vi "Read Recordset (STRING).vi"(8 "error in (no error)":errorcluster, 9 "Max Rows to Fetch (-1 = all)":i32=-1, 11 "Recordset In":refnum<k7>) -> (0 "error out":errorcluster, 1 "Rows Returned":i32, 2 "Data out":string[][](array[string]), 3 "Recordset Out":refnum<k7>, 4 "Field Names":string[](array[string]))   [LabVIEW 2014, in "hse-db.lvlib" / "ADO-DB-Driver.lvlib"]
uses:
  ADO-DB-Driver.lvlib
panel:
  out "records read so far":i32
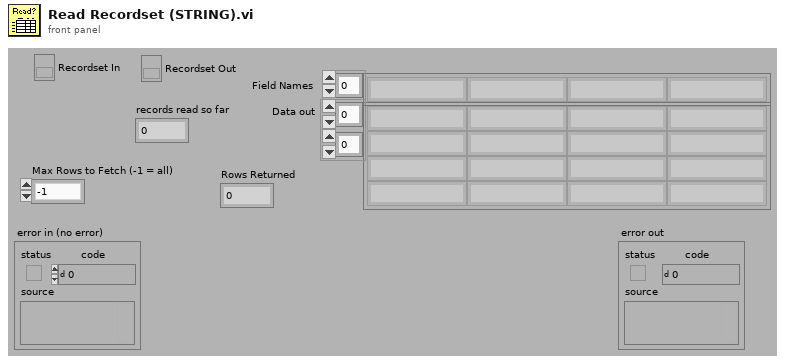
[diagram p1: front panel]
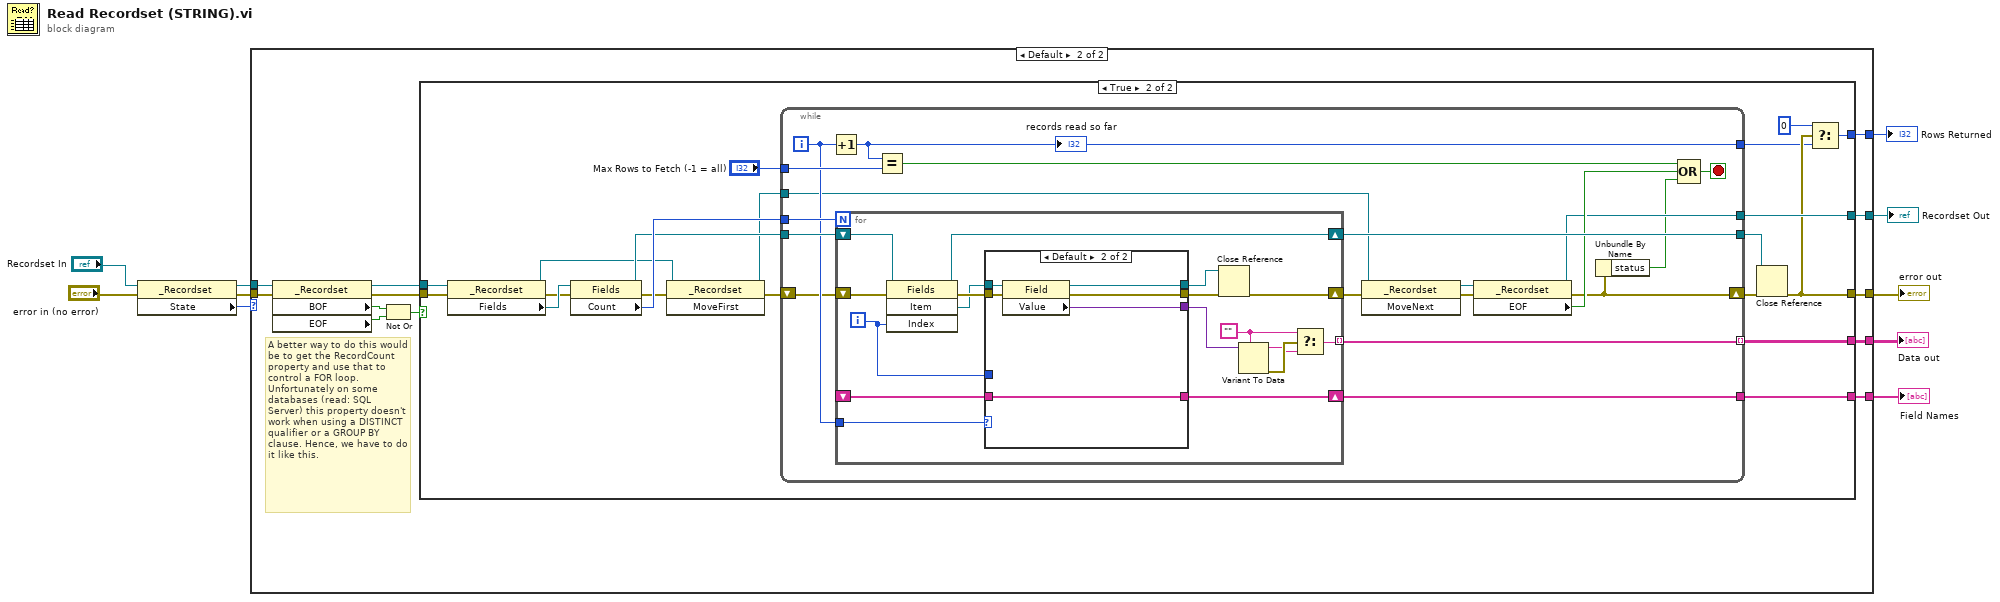
[diagram p0: block diagram]
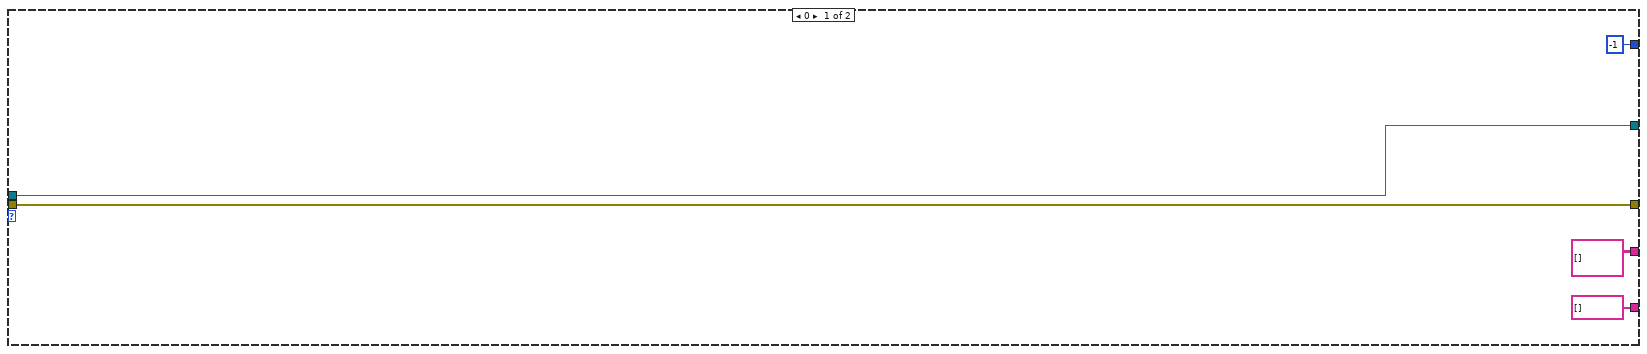
[diagram p2: hidden frame]
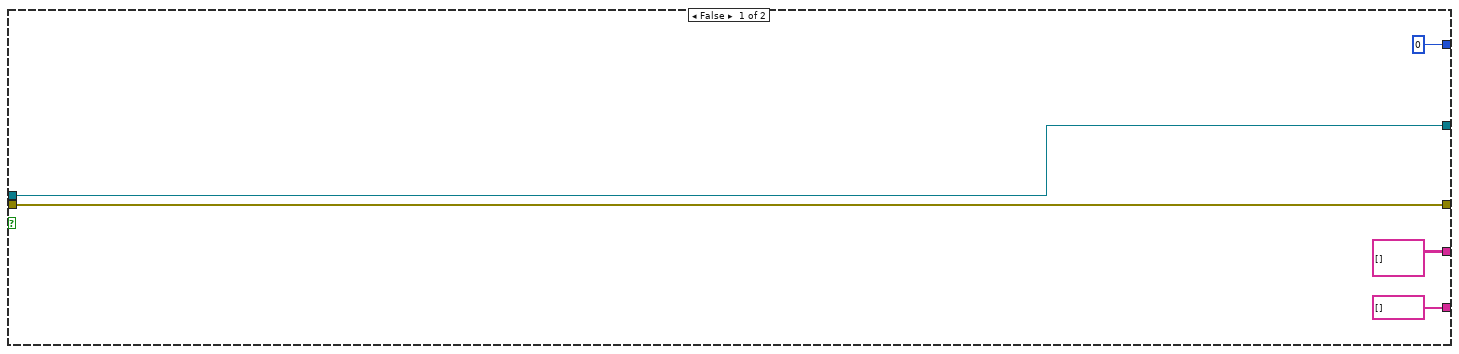
[diagram p3: hidden frame]
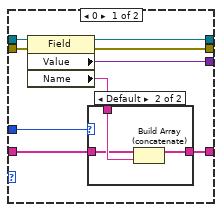
[diagram p4: hidden frame]
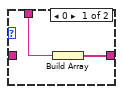
[diagram p5: hidden frame]
diagram:
  n1 = property class="_Recordset"(reference="Recordset In", error in="error in (no error)") -> (reference out=w5:refnum<k7>, error out=w3:errorcluster, "State"=w2:i32)
  n2 = case shown="Default" w2 {
    tunnel: [string[][] [] w27] -> w10
    tunnel: [w11 w26] -> w9
    tunnel: [string[] [] w25] -> w8
    tunnel: [w15 w22] -> w1
    tunnel: [-1 w21] -> w7
    tunnel: w5 -> [w11 w17]
    tunnel: w3 -> [w15 w16]
    frame 0 {
    }
    frame Default {
      # "A better way to do this would be to get the RecordCount property and use that to control a FOR loop. Unfortunately on some databases (read: SQL Server) this property doesn't work when using a DISTINCT qualifier or a GROUP BY clause. Hence, we have to do it like this."
      n3 = property class="_Recordset"(reference=w17, error in=w16) -> (reference out=w24:refnum<k7>, error out=w23:errorcluster, "BOF"=w20:bool, "EOF"=w18:bool)
      n4 = Not Or(1:w18, 2:w20) -> (0:w19:bool)
      n5 = case shown="True" w19 {
        tunnel: [string[][] [] w48] -> w27
        tunnel: [w32 w52] -> w26
        tunnel: [string[] [] w49] -> w25
        tunnel: w24 -> [w32 w51]
        tunnel: w23 -> [w31 w50]
        tunnel: [w31 w46] -> w22
        tunnel: [0 ("Rows Returned") w47] -> w21
        frame False {
        }
        frame True {
          n6 = property class="_Recordset"(reference=w51, error in=w50) -> (reference out=w34:refnum<k7>, error out=w44:errorcluster, "Fields"=w45:refnum<k7>)
          n7 = property class="Fields"(reference=w45, error in=w44) -> (reference out=w39:refnum<k7>, error out=w37:errorcluster, "Count"=w43:i32)
          n8 = invoke class="_Recordset" method="MoveFirst"(reference=w34, error in=w37) -> (reference out=w36:refnum<k7>, error out=w35:errorcluster)  [unwired: 1 in, 1 out]
          n9 = while {
            shift-right: [w53] -> w42
            shift-left: w35 -> [w58]
            tunnel: [w71] -> w48 mode=indexing
            tunnel: w43 -> [w70]
            tunnel: "Max Rows to Fetch (-1 = all)" -> [w66]
            tunnel: [w61] -> w41
            tunnel: [w63] -> w49
            tunnel: w36 -> [w59]
            tunnel: [w55] -> w52
            tunnel: w39 -> [w69]
            tunnel: [w68] -> w38
            i -> [w64]
            stop <- w67 stop-if-true
            n10 = Increment(x=w64) -> (x+1=w61:i32)
            "records read so far" <- w61
            n11 = for {
              N: w70 -> [_]
              shift-right: [w82] -> w60
              shift-left: w58 -> [w87]
              tunnel: [w78] -> w71 mode=indexing
              shift-right: [w83] -> w68
              shift-left: w69 -> [w84]
              tunnel: w64 -> [w75]
              shift-right: [w73] -> w63
              shift-left: _ -> [w74]
              i -> [w72]
              w77 = ""
              n12 = invoke class="Fields" method="Item"(reference=w84, error in=w87, "Index"=w72) -> (reference out=w83:refnum<k7>, error out=w88:errorcluster, "Item"=w76:refnum<k7>)  [unwired: 1 in, 1 out]
              n13 = case shown="Default" w75 {
                tunnel: w88 -> [w97 w108]
                tunnel: [w96 w105] -> w86
                tunnel: [w95 w106] -> w85
                tunnel: [w94 w104] -> w81
                tunnel: w76 -> [w93 w107]
                tunnel: w72 -> [w92 _]
                tunnel: w74 -> [w91 w103]
                tunnel: [w90 w103] -> w73
                frame 0 {
                  n14 = property class="Field"(reference=w93, error in=w97) -> (reference out=w96:refnum<k7>, error out=w95:errorcluster, "Value"=w94:variant, "Name"=w89:string)
                  n15 = case shown="Default" w92 {
                    tunnel: w91 -> [_ w101]
                    tunnel: [w98 w100] -> w90
                    tunnel: w89 -> [w99 w102]
                    frame 0 {
                      n16 = Build Array(w99) -> (w98:string[])
                    }
                    frame Default {
                      n17 = Build Array (concatenate)(w101, w102) -> (w100:string[])
                    }
                  }
                }
                frame Default {
                  n18 = property class="Field"(reference=w107, error in=w108) -> (reference out=w105:refnum<k7>, error out=w106:errorcluster, "Value"=w104:variant)
                }
              }
              n19 = Close Reference(reference=w86, error in (no error)=w85) -> (error out=w82:errorcluster)
              n20 = Variant To Data(type=w77, Variant=w81) -> (data=w79:string, error out=w80:errorcluster)  [unwired: 1 in]
              n21 = Select(t=w77, s=w80, f=w79) -> (s? t:f=w78:string)
            }
            n22 = Equal?(x=w61, y=w66) -> (x = y?=w65:bool)
            n23 = invoke class="_Recordset" method="MoveNext"(reference=w59, error in=w60) -> (reference out=w57:refnum<k7>, error out=w56:errorcluster)  [unwired: 1 in, 1 out]
            n24 = property class="_Recordset"(reference=w57, error in=w56) -> (reference out=w55:refnum<k7>, error out=w53:errorcluster, "EOF"=w62:bool)
            n25 = Unbundle By Name(w53) -> ("status"=w54:bool)
            n26 = Compound Arithmetic op=OR(w65, w62, w54) -> (w67:bool)
          }
          n27 = Close Reference(reference=w38, error in (no error)=w42) -> (error out=w46:errorcluster)
          n28 = Select(t=0, s=w46, f=w41) -> (s? t:f=w47:i32)
        }
      }
    }
  }
  "Data out" <- w10
  "error out" <- w1
  "Rows Returned" <- w7
  "Recordset Out" <- w9
  "Field Names" <- w8
